vi "Destroy.vi"(8 "Error In":errorcluster, 11 "NI9862 in":refnum<class "NI9862.lvclass">) -> (0 "Error Out":errorcluster, 3 "NI9862 out":refnum<class "NI9862.lvclass">)   [LabVIEW 2024, in "NI9862.lvclass"]
uses:
  NI9862.lvclass/NI9862.ctl
  NI9862.lvclass
  Source/Interfaces/IInstrument/IInstrument.lvclass
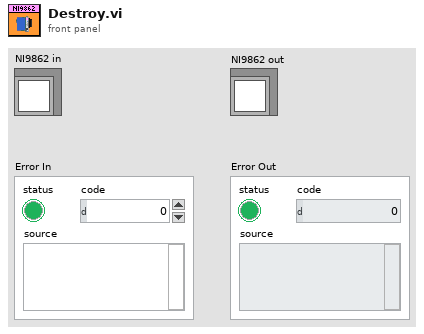
[diagram p1: front panel]
types:
  T1 = typedef "NI9862.lvclass/ObjectAttributes.ctl" = cluster{"IConfigure":refnum<class "IConfigure.lvclass">}
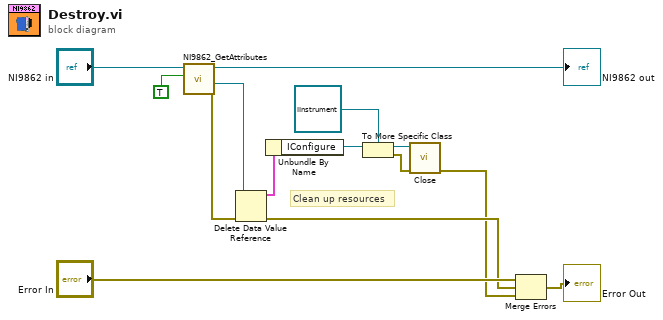
[diagram p0: block diagram]
diagram:
  # "Clean up resources"
  n1 = call "NI9862_GetAttributes.vi"("OnlyGetDvrReference(False)"=TRUE, "NI9862 in"="NI9862 in") -> ("Error Out"=w11:errorcluster, "DataRef"=w10:refnum<data-value>, "NI9862 out"=→"NI9862 out":refnum<class "NI9862.lvclass">)  [unwired: 6 in, 1 out]
  n2 = Delete Data Value Reference(data value reference=w10, error in=w11) -> (data value=w7:T1, error out=w2:errorcluster)
  n3 = Unbundle By Name(w7) -> ("IConfigure"=w6:refnum<class "IConfigure.lvclass">)
  n4 = To More Specific Class(target class=refnum<class "IInstrument.lvclass"> refnum ("IInstrument.lvclass"), reference=w6) -> (specific class reference=w3:refnum<class "IInstrument.lvclass">, error out=w4:errorcluster)  [unwired: 1 in]
  n5 = call-dynamic "Close.vi"("error in"=w4, "IInstrument in"=w3) -> ("error out"=w1:errorcluster)  [unwired: 8 in, 1 out]
  n6 = Merge Errors("Error In", w2, w1) -> (→"Error Out":errorcluster)
